vi "Robot-centric button movement.vi"(10 "Cluster":T2, 11 "Drive Controls":T1) -> (3 "Drive Out":T1)   [LabVIEW 2014]
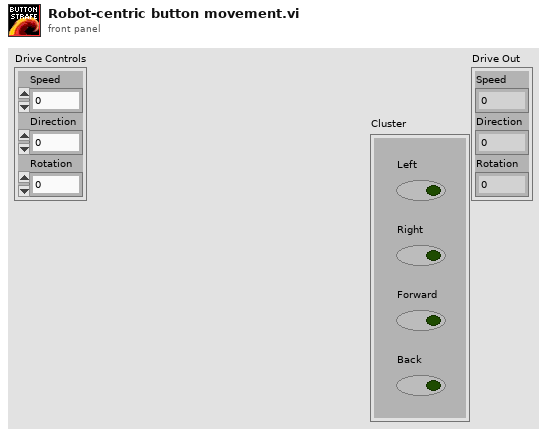
[diagram p1: front panel]
types:
  T1 = cluster{"Speed":dbl, "Direction":dbl, "Rotation":dbl}
  T2 = cluster{"Left":bool, "Right":bool, "Forward":bool, "Back":bool}
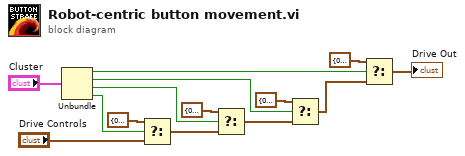
[diagram p0: block diagram]
diagram:
  n1 = Unbundle("Cluster") -> ("Left"=w7:bool, "Right"=w8:bool, "Forward"=w9:bool, "Back"=w10:bool)
  n2 = Select(t=T1 {"Speed"=0.25, "Direction"=3.14159, "Rotation"=0.0} ("Drive Controls"), s=w10, f="Drive Controls") -> (s? t:f=w14:T1)
  n3 = Select(t=T1 {"Speed"=0.25, "Direction"=0.0, "Rotation"=0.0} ("Drive Controls"), s=w9, f=w14) -> (s? t:f=w13:T1)
  n4 = Select(t=T1 {"Speed"=0.25, "Direction"=4.712385, "Rotation"=0.0} ("Drive Controls"), s=w8, f=w13) -> (s? t:f=w12:T1)
  n5 = Select(t=T1 {"Speed"=0.25, "Direction"=1.570795, "Rotation"=0.0} ("Drive Controls"), s=w7, f=w12) -> (s? t:f=→"Drive Out":T1)
